vi "GetScopeBrdcstEvents.vi"(7 "error in (no error)":errorcluster) -> (3 "Event Registration Refnum":refnum<event-registration>, 5 "error out":errorcluster)   [LabVIEW 2018, in "Test.lvclass"]
uses:
  Test.lvclass
  Scope/ScopeModule/Protected/clEventType.ctl
  Scope/ScopeModule/ScopeModule.lvlib
  Scope/ScopeShared/ScopeShared.lvlib
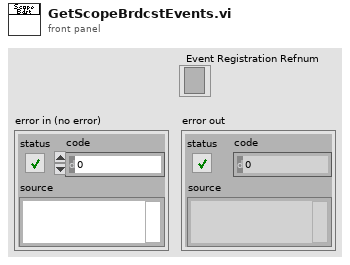
[diagram p1: front panel]
types:
  T1 = typedef "ScopeShared.lvlib/clBroadcastEvents.ctl" = cluster{"DidInit":refnum<user-event>, "StatusUpdate":refnum<user-event>, "ErrorReport":refnum<user-event>, "DidStop":refnum<user-event>, "PathToINI":refnum<user-event>, "Handle":refnum<user-event>, "Model":refnum<user-event>, "Channels":refnum<user-event>, "Acquisition":refnum<user-event>, "Trigger":refnum<user-event>, "ExtAcquisition":refnum<user-event>, "Waveform":refnum<user-event>}
  T2 = cluster{"Acquisition":refnum<user-event>, "Channels":refnum<user-event>, "Trigger":refnum<user-event>, "Waveform":refnum<user-event>, "ErrorReport":refnum<user-event>}
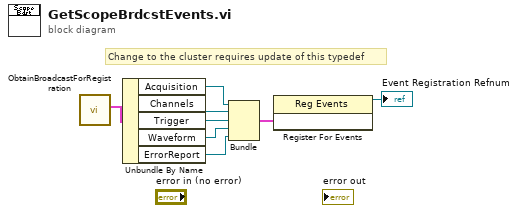
[diagram p0: block diagram]
diagram:
  # "Change to the cluster requires update of this typedef"
  n1 = call "ObtainBroadcastForRegistration.vi"() -> ("clBroadcastEvents"=w8:T1)  [unwired: 10 in, 1 out]
  n2 = Unbundle By Name(w8) -> ("Acquisition"=w7:refnum<user-event>, "Channels"=w6:refnum<user-event>, "Trigger"=w5:refnum<user-event>, "Waveform"=w3:refnum<user-event>, "ErrorReport"=w2:refnum<user-event>)
  n3 = Bundle("Acquisition"=w7, "Channels"=w6, "Trigger"=w5, "Waveform"=w3, "ErrorReport"=w2) -> (w4:T2)  [unwired: 1 in]
  n4 = register-events(w4) -> (reference out=→"Event Registration Refnum":refnum<event-registration>)  [unwired: 2 in, 1 out]
